vi "UI Subpanel.vi"() -> ()   [LabVIEW 2021, in "CIF Template UI.lvlib"]
uses:
  CIF Template UI.lvlib
  Common/Typedef/Configuration.ctl
  <vilib>/CIF Foundation/CIF Core/CIFCore/Common/Typedef/Common Plugin Configuration.ctl
  <vilib>/CIF Foundation/CIF Core/CIFUI/Typedef/Class Data for SubPanel.ctl
  <vilib>/gRPC/LabVIEW gRPC Library/Shared/grpcId.ctl
  <vilib>/CIF Foundation/CIF Core/CIFUI/Typedef/Core UI References.ctl
  <vilib>/CIF Foundation/CIF Core/CIFUI/Typedef/Channel Connection.ctl
  <vilib>/CIF Foundation/CIF Core/CIFUI/Typedef/New Plugin.ctl
  <vilib>/CIF Foundation/CIF Core/CIFUI/Typedef/Run Listen Button.ctl
  <vilib>/CIF Foundation/CIF Core/CIFUI/Typedef/CIF_Manager_UI_Tab.ctl
  <vilib>/CIF Foundation/CIF Core/CIFUI/Typedef/SubPanel Events.ctl
  <vilib>/CIF Foundation/CIF Core/CIFUI/Typedef/New Connection Event Data.ctl
  <vilib>/CIF Foundation/CIF Core/CIFUI/Typedef/New Connection Plugin Event Data.ctl
  <vilib>/CIF Foundation/CIF Core/CIFUI/CIF_UI.lvclass
  <vilib>/CIF Foundation/CIF Core/CIFUI/CIF_UI.lvclass/CIF_UI.ctl
  <vilib>/CIF Foundation/CIF Core/CIFUI/Utilities/Get Human Readable Error.vi
  <vilib>/CIF Foundation/CIF Utilities/Errors/Human Readable Error Message.vi
  Grpc/Template_wrapper/Template_Wrapper.lvlib
  <vilib>/addons/_JKI.lib/Serialization/JSON/JKI JSON Serialization.lvlib
  <vilib>/CIF Foundation/CIF Core/CIFCore/Grpc/CIFCoreWrapper/CIFCoreWrapper.lvlib
  <vilib>/CIF Foundation/CIF Core/CIFCore/Common/CIFCoreCommon.lvlib
  Common/Template_Common.lvlib
  <vilib>/gRPC/LabVIEW gRPC Library/grpc-lvsupport-release.lvlib
panel:
  in  "Class Data for SubPanel":T1
  in  "Update Config":bool
  in  "Configuration":T5={"Common"={"Period (s)"=0.001, "Offset (us)"=0, "ClockID"=0, "Priority"=100, "Processor"=-2}, "Step"=100} {"Common"."Period (s)" format="%#_13g"}
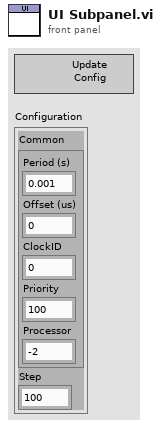
[diagram p1: front panel]
types:
  T1 = typedef "CIF_UI.lvclass/Class Data for SubPanel.ctl" = cluster{"IP Address":string, "Manager gRPC ID":T2, "Server Certificate File (.crt)":path, "Connected":bool, "Manager Connection":bool, "Core UI References":T3, "Subpanel Events":T4}
  T2 = typedef "grpc-lvsupport-release.lvlib/grpcId.ctl" = u64
  T3 = typedef "CIF_UI.lvclass/Core UI References.ctl" = cluster{"Discovered Plugins":refnum<vi>, "Discovered Plugins Valid":bool, "Loaded Plugins":refnum<vi>, "Loaded Plugins Valid":bool, "Publisher Channels":refnum<vi>, "Publisher Channels Valid":bool, "Subscriber Channels":refnum<vi>, "Subscriber Channels Valid":bool, "Plugin Status":refnum<vi>, "Plugin Status Valid":bool, "Channel Connection":refnum<vi>, "Channel Connection Valid":bool, "New Plugin Load":refnum<vi>, "New Plugin Load Valid":bool, "Errors":refnum<vi>, "Errors Valid":bool, "Plugin to Abort":refnum<vi>, "Plugin to Abort Valid":bool, "Connection":refnum<vi>, "Connection Valid":bool, "Exit":refnum<vi>, "Exit Valid":bool, "Run Listen":refnum<vi>, "Run Listen Valid":bool, "CIF Manager Tab":refnum<vi>, "Manger Tab Valid":bool, "Clear Local Error":refnum<vi>, "Clear Local Error Valid":bool, "Local Error":refnum<vi>, "Local Error Valid":bool, "System Errors":refnum<vi>, "System Errors Valid":bool, "Plugin Selection":refnum<vi>, "Plugin Selection Valid":bool}
  T4 = typedef "CIF_UI.lvclass/SubPanel Events.ctl" = cluster{"Clear Local Error":refnum<user-event>, "Shutdown":refnum<user-event>, "gRPC Connection":refnum<user-event>, "Plugin Connection":refnum<user-event>}
  T5 = typedef "Template_Common.lvlib/Configuration.ctl" = cluster{"Common":T6, "Step":u64}
  T6 = typedef "CIFCoreCommon.lvlib/Common Plugin Configuration.ctl" = cluster{"Period (s)":dbl, "Offset (us)":i32, "ClockID":u8, "Priority":i32, "Processor":i32}
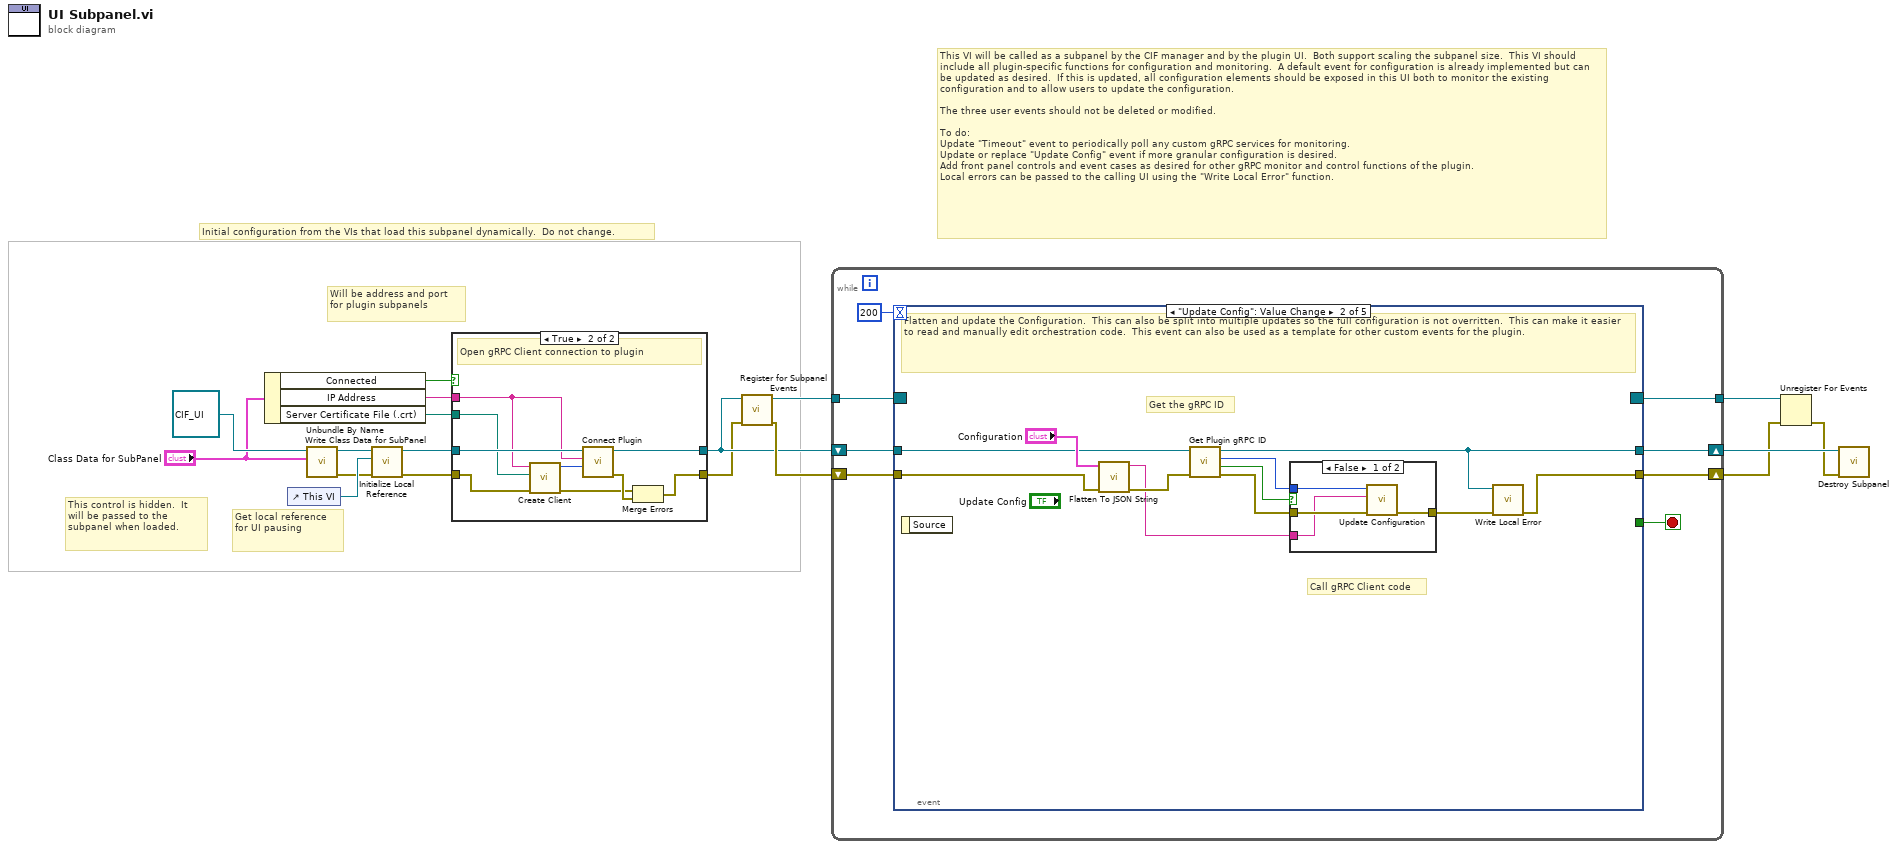
[diagram p0: block diagram]
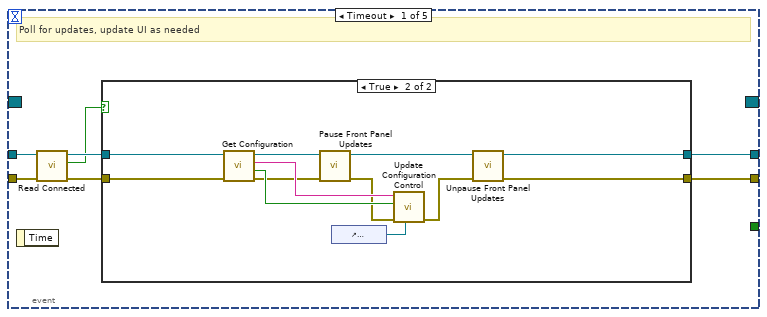
[diagram p3: hidden frame]
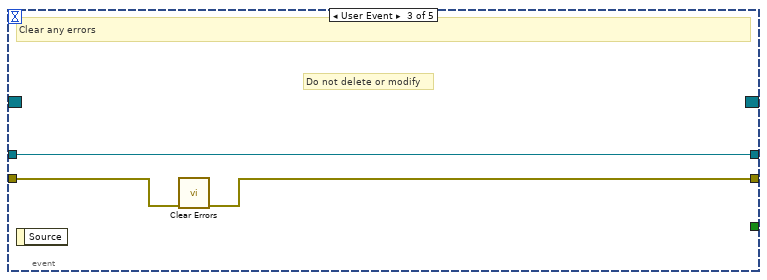
[diagram p6: hidden frame]
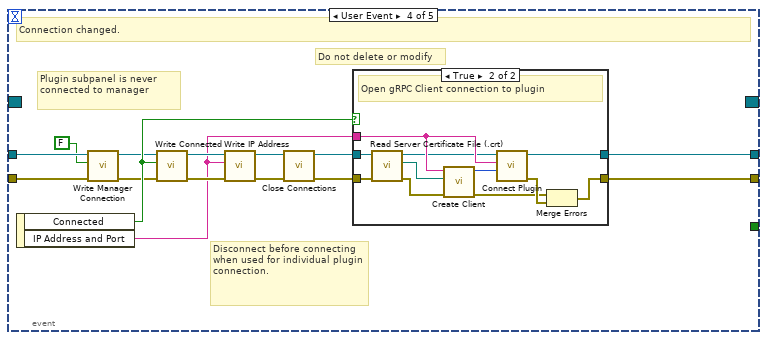
[diagram p7: hidden frame]
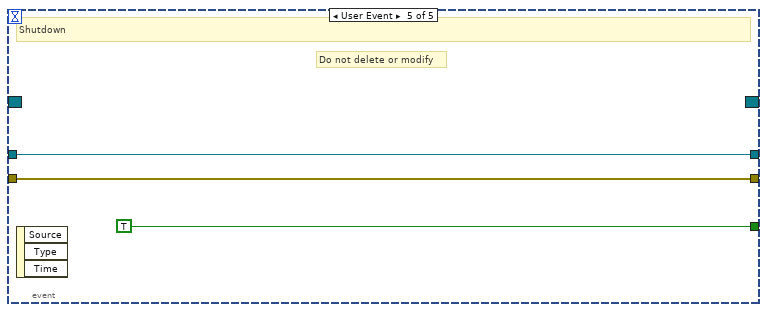
[diagram p9: hidden frame]
diagram:
  # "Initial configuration from the VIs that load this subpanel dynamically.  Do not change."
  # "This control is hidden.  It will be passed to the subpanel when loaded."
  # "This VI will be called as a subpanel by the CIF manager and by the plugin UI.  Both support scaling the subpanel size.  This VI should include all plugin-specific functions for configuration and monitoring.  A default event for configuration is already implemented but can be updated as desired.  If this is updated, all configuration elements should be exposed in this UI both to monitor the existing configuration and to allow users to update the configuration.\n\nThe three user events should not be deleted or modified.\n\nTo do:\nUpdate \"Timeout\" event to periodically poll any custom gRPC services for monitoring.\nUpdate or replace \"Update Config\" event if more granular configuration is desired.\nAdd front panel controls and event cases as desired for other gRPC monitor and control functions of the plugin.\nLocal errors can be passed to the calling UI using the \"Write Local Error\" function."
  # "Will be address and port for plugin subpanels"
  # "Get local reference for UI pausing"
  n1 = Unbundle By Name("Class Data for SubPanel") -> ("Connected"=w3:bool, "IP Address"=w2:string, "Server Certificate File (.crt)"=w1:path)
  n2 = control-ref of="This VI"() -> (w18:refnum<vi>)
  n3 = call <vilib>:"Write Class Data for SubPanel.vi"("Class Data for SubPanel"="Class Data for SubPanel", "CIF_UI in"=refnum<class "CIF_UI.lvclass"> refnum) -> ("error out"=w9:errorcluster, "CIF_UI out"=w11:refnum<class "CIF_UI.lvclass">)  [unwired: 8 in]
  n4 = call <vilib>:"Initialize Local Reference.vi"("error in (no error)"=w9, "This VI"=w18, "CIF_UI in"=w11) -> ("error out"=w7:errorcluster, "CIF_UI out"=w8:refnum<class "CIF_UI.lvclass">)  [unwired: 7 in]
  n5 = case shown="True" w3 {
    tunnel: [w19 w29] -> w5
    tunnel: [w20 w27] -> w6
    tunnel: w8 -> [w20 w26]
    tunnel: w7 -> [w19 w25]
    tunnel: w2 -> [_ w22]
    tunnel: w1 -> [_ w21]
    frame False {
    }
    frame True {
      # "Open gRPC Client connection to plugin"
      n6 = call "Create Client.vi"("error in"=w25, "Server Certificate File (.crt)"=w21, "address"=w22) -> ("error out"=w24:errorcluster, "gRPC ID Out"=w23:T2)  [unwired: 7 in]
      n7 = call <vilib>:"Connect Plugin.vi"("gRPC ID"=w23, "Address"=w22, "CIF_UI in"=w26) -> ("error out"=w28:errorcluster, "CIF_UI out"=w27:refnum<class "CIF_UI.lvclass">)  [unwired: 7 in]
      n8 = Merge Errors(w24, w28) -> (w29:errorcluster)
    }
  }
  n9 = call <vilib>:"Register for Subpanel Events.vi"("error in (no error)"=w5, "CIF_UI in"=w6) -> ("error out"=w16:errorcluster, "Event Registration Refnum"=w17:refnum<event-registration>)  [unwired: 8 in]
  n10 = while {
    tunnel: w17 -> [w36]
    shift-right: [w31] -> w15
    shift-left: w6 -> [w34]
    shift-right: [w32] -> w13
    shift-left: w16 -> [w33]
    tunnel: [w30] -> w14
    stop <- w35 stop-if-true
    n11 = event shown="[1] \"Update Config\": Value Change" {
      selector: w36 -> [_ _ _ _ _]
      dyn-events: [_ _ _ _ _] -> w30
      timeout: 200 -> [_ _ _ _ _]
      tunnel: [_ _ _ _ TRUE] -> w35
      tunnel: w34 -> [w40 w64 w75 w82 w107]
      tunnel: w33 -> [w41 w68 w77 w81 w106]
      tunnel: [w38 w60 w76 w83 w106] -> w32
      tunnel: [w39 w59 w75 w84 w107] -> w31
      event Timeout {
        # "Poll for updates, update UI as needed"
        n12 = event-data() -> ()  [unwired: 1 in, 1 out]
        n13 = call <vilib>:"Read Connected.vi"("error in (no error)"=w41, "CIF_UI in"=w40) -> ("error out"=w43:errorcluster, "Connected"=w42:bool, "CIF_UI out"=w44:refnum<class "CIF_UI.lvclass">)  [unwired: 7 in]
        n14 = case shown="True" w42 {
          tunnel: w43 -> [w45 w51]
          tunnel: [w45 w58] -> w38
          tunnel: w44 -> [w46 w52]
          tunnel: [w46 w57] -> w39
          frame False {
          }
          frame True {
            n15 = call <vilib>:"Get Configuration.vi"("error in (no error)"=w51, "CIF_Plugin_UI in"=w52) -> ("error out"=w49:errorcluster, "Not Found"=w54:bool, "JSON Configuration"=w55:string, "CIF_Plugin_UI out"=w50:refnum<class "CIF_UI.lvclass">)  [unwired: 6 in]
            n16 = call <vilib>:"Pause Front Panel Updates.vi"("error in (no error)"=w49, "CIF_UI in"=w50) -> ("error out"=w48:errorcluster, "CIF_UI out"=w47:refnum<class "CIF_UI.lvclass">)  [unwired: 8 in]
            n17 = control-ref of="Configuration"() -> (w53:refnum<vi>)
            n18 = call "Update Configuration Control.vi"("Configuration reference"=w53, "error in (no error)"=w48, "Not Valid"=w54, "JSON Configuration"=w55) -> ("error out"=w56:errorcluster)  [unwired: 7 in]
            n19 = call <vilib>:"Unpause Front Panel Updates.vi"("error in (no error)"=w56, "CIF_UI in"=w47) -> ("error out"=w58:errorcluster, "CIF_UI out"=w57:refnum<class "CIF_UI.lvclass">)  [unwired: 8 in]
          }
        }
      }
      event "Update Config": Value Change {
        # "Call gRPC Client code"
        # "Get the gRPC ID"
        # "Flatten and update the Configuration.  This can also be split into multiple updates so the full configuration is not overritten.  This can make it easier to read and manually edit orchestration code.  This event can also be used as a template for other custom events for the plugin."
        n20 = event-data() -> ()  [unwired: 1 in, 1 out]
        n21 = call <vilib>:"Flatten To JSON String.vi"("error in (no error)"=w68, "Variant"="Configuration") -> ("error out"=w63:errorcluster, "JSON String"=w62:string)  [unwired: 8 in]
        n22 = call <vilib>:"Get Plugin gRPC ID.vi"("error in (no error)"=w63, "CIF_UI in"=w64) -> ("error out"=w65:errorcluster, "Not Found"=w66:bool, "gRPC ID"=w67:T2, "CIF_UI out"=w59:refnum<class "CIF_UI.lvclass">)  [unwired: 5 in, 1 out]
        n23 = case shown="False" w66 {
          tunnel: w67 -> [w73 _]
          tunnel: w65 -> [w72 w74]
          tunnel: [w71 w74] -> w61
          tunnel: w62 -> [w70 _]
          frame False {
            n24 = call <vilib>:"Update Configuration.vi"("error in"=w72, "JSON Configuration"=w70, "gRPC ID"=w73) -> ("error out"=w71:errorcluster)  [unwired: 7 in, 1 out]
          }
          frame True {
          }
        }
        n25 = call <vilib>:"Write Local Error.vi"("error in (no error)"=w61, "CIF_UI in"=w59) -> ("error out"=w60:errorcluster)  [unwired: 9 in]
      }
      event User Event {
        # "Do not delete or modify"
        # "Clear any errors"
        n26 = event-data() -> ()  [unwired: 1 in, 1 out]
        n27 = call <vilib>:"Clear Errors.vi"("error in (no error)"=w77) -> ("error out"=w76:errorcluster)  [unwired: 5 in, 1 out]
      }
      event User Event {
        # "Do not delete or modify"
        # "Plugin subpanel is never connected to manager"
        # "Disconnect before connecting when used for individual plugin connection."
        # "Connection changed."
        n28 = event-data() -> ("Connected"=w85:bool, "IP Address and Port"=w86:string)  [unwired: 1 in]
        n29 = call <vilib>:"Write Manager Connection.vi"("error in (no error)"=w81, "Manager Connection"=FALSE, "CIF_UI in"=w82) -> ("error out"=w79:errorcluster, "CIF_UI out"=w80:refnum<class "CIF_UI.lvclass">)  [unwired: 7 in]
        n30 = call <vilib>:"Write Connected.vi"("error in (no error)"=w79, "Connected"=w85, "CIF_UI in"=w80) -> ("error out"=w91:errorcluster, "CIF_UI out"=w92:refnum<class "CIF_UI.lvclass">)  [unwired: 7 in]
        n31 = call <vilib>:"Write IP Address.vi"("error in (no error)"=w91, "IP Address"=w86, "CIF_UI in"=w92) -> ("error out"=w89:errorcluster, "CIF_UI out"=w90:refnum<class "CIF_UI.lvclass">)  [unwired: 7 in]
        n32 = call <vilib>:"Close Connections.vi"("error in (no error)"=w89, "CIF_UI in"=w90) -> ("error out"=w87:errorcluster, "CIF_UI out"=w88:refnum<class "CIF_UI.lvclass">)  [unwired: 8 in]
        n33 = case shown="True" w85 {
          tunnel: [w93 w105] -> w83
          tunnel: [w94 w103] -> w84
          tunnel: w88 -> [w94 w99]
          tunnel: w87 -> [w93 w98]
          tunnel: w86 -> [_ w100]
          frame False {
          }
          frame True {
            # "Open gRPC Client connection to plugin"
            n34 = call <vilib>:"Read Server Certificate File (.crt).vi"("error in (no error)"=w98, "CIF_UI in"=w99) -> ("error out"=w96:errorcluster, "Server Certificate File (.crt)"=w95:path, "CIF_UI out"=w97:refnum<class "CIF_UI.lvclass">)  [unwired: 7 in]
            n35 = call "Create Client.vi"("error in"=w96, "Server Certificate File (.crt)"=w95, "address"=w100) -> ("error out"=w102:errorcluster, "gRPC ID Out"=w101:T2)  [unwired: 7 in]
            n36 = call <vilib>:"Connect Plugin.vi"("gRPC ID"=w101, "Address"=w100, "CIF_UI in"=w97) -> ("error out"=w104:errorcluster, "CIF_UI out"=w103:refnum<class "CIF_UI.lvclass">)  [unwired: 7 in]
            n37 = Merge Errors(w102, w104) -> (w105:errorcluster)
          }
        }
      }
      event User Event {
        # "Do not delete or modify"
        # "Shutdown"
        n38 = event-data() -> ()  [unwired: 1 in, 3 out]
      }
    }
  }
  n39 = Unregister For Events(event registration refnum=w14, error in=w13) -> (error out=w12:errorcluster)
  n40 = call <vilib>:"Destroy Subpanel.vi"("error in (no error)"=w12, "CIF_UI in"=w15) -> ()  [unwired: 8 in, 2 out]
